vi "HFRR ADV v07 new software.vi"() -> ()   [LabVIEW 2025] (continued)
        n796 = local write "LIVE FEED MAX TEMP"(TRUE ("LIVE FEED MAX TEMP")) -> ()
        n797 = case shown="True" w1177 {
          selector: w1177 -> [_ w1186]
          frame False {
          }
          frame True {
            n798 = Not(x=w1186) -> (.not. x?=w1185:bool)
            n799 = local write "LIVE FEED MIN TEMP"(w1185) -> ()
            n800 = call "CAMERA LIVE FEED FGV.vi"("Enum - Menu"=CAMERA_LIVE_FEED_ENUM."CAMERA MINIMIZE") -> ()  [unwired: 9 in, 2 out]
          }
        }
        n801 = case shown="True" w1175 {
          selector: w1175 -> [_ w1183]
          frame False {
          }
          frame True {
            n802 = Not(x=w1183) -> (.not. x?=w1181:bool)
            n803 = local write "CAMERA ROI MAX TEMP"(w1181) -> ()
            n804 = call "IMAGE ANALYSIS.vi"("Enum"=POST_ANALYSIS_ENUM."SHOW UI") -> ("error out"=w1180:errorcluster)  [unwired: 9 in, 1 out]
            n805 = call "LIST FILE NAMES.vi"("error in (no error)"=w1180) -> ("filenames"=w1179:string[])  [unwired: 9 in, 1 out]
            n806 = property on="Test File List :" class="CmbBox"("Strings[]"=w1179) -> ()  [unwired: 2 in, 2 out]
          }
        }
        n807 = local write "CAMERA ROI MIN TEMP"(TRUE ("CAMERA ROI MIN TEMP")) -> ()
      }
      frame "Compare Files" {
        n808 = local read "LIVE FEED MIN TEMP"() -> (w1189:bool)
        n809 = local write "LIVE FEED MAX TEMP"(TRUE ("LIVE FEED MAX TEMP")) -> ()
        n810 = local read "CAMERA ROI MIN TEMP"() -> (w1187:bool)
        n811 = case shown="True" w1189 {
          selector: w1189 -> [_ w1196]
          frame False {
          }
          frame True {
            n812 = Not(x=w1196) -> (.not. x?=w1195:bool)
            n813 = local write "LIVE FEED MIN TEMP"(w1195) -> ()
            n814 = call "CAMERA LIVE FEED FGV.vi"("Enum - Menu"=CAMERA_LIVE_FEED_ENUM."CAMERA MINIMIZE") -> ()  [unwired: 9 in, 2 out]
          }
        }
        n815 = case shown="True" w1187 {
          selector: w1187 -> [_ w1193]
          frame False {
          }
          frame True {
            n816 = Not(x=w1193) -> (.not. x?=w1192:bool)
            n817 = local write "CAMERA ROI MIN TEMP"(w1192) -> ()
            n818 = call "IMAGE ANALYSIS.vi"("Enum"=POST_ANALYSIS_ENUM."MINIMIZE UI") -> ()  [unwired: 9 in, 2 out]
          }
        }
        n819 = local write "CAMERA ROI MAX TEMP"(TRUE ("CAMERA ROI MAX TEMP")) -> ()
      }
      frame "About" {
        n820 = local read "LIVE FEED MIN TEMP"() -> (w1199:bool)
        n821 = local write "LIVE FEED MAX TEMP"(TRUE ("LIVE FEED MAX TEMP")) -> ()
        n822 = local read "CAMERA ROI MIN TEMP"() -> (w1198:bool)
        n823 = case shown="True" w1199 {
          selector: w1199 -> [_ w1206]
          frame False {
          }
          frame True {
            n824 = Not(x=w1206) -> (.not. x?=w1205:bool)
            n825 = local write "LIVE FEED MIN TEMP"(w1205) -> ()
            n826 = call "CAMERA LIVE FEED FGV.vi"("Enum - Menu"=CAMERA_LIVE_FEED_ENUM."CAMERA MINIMIZE") -> ()  [unwired: 9 in, 2 out]
          }
        }
        n827 = case shown="True" w1198 {
          selector: w1198 -> [_ w1203]
          frame False {
          }
          frame True {
            n828 = Not(x=w1203) -> (.not. x?=w1202:bool)
            n829 = local write "CAMERA ROI MIN TEMP"(w1202) -> ()
            n830 = call "IMAGE ANALYSIS.vi"("Enum"=POST_ANALYSIS_ENUM."MINIMIZE UI") -> ()  [unwired: 9 in, 2 out]
          }
        }
        n831 = local write "CAMERA ROI MAX TEMP"(TRUE ("CAMERA ROI MIN TEMP")) -> ()
      }
      frame "Advance" {
        n832 = local read "LIVE FEED MIN TEMP"() -> (w1209:bool)
        n833 = local write "LIVE FEED MAX TEMP"(TRUE ("LIVE FEED MAX TEMP")) -> ()
        n834 = local read "CAMERA ROI MIN TEMP"() -> (w1207:bool)
        n835 = case shown="True" w1209 {
          selector: w1209 -> [_ w1216]
          frame False {
          }
          frame True {
            n836 = Not(x=w1216) -> (.not. x?=w1215:bool)
            n837 = local write "LIVE FEED MIN TEMP"(w1215) -> ()
            n838 = call "CAMERA LIVE FEED FGV.vi"("Enum - Menu"=CAMERA_LIVE_FEED_ENUM."CAMERA MINIMIZE") -> ()  [unwired: 9 in, 2 out]
          }
        }
        n839 = local write "CAMERA ROI MAX TEMP"(TRUE ("CAMERA ROI MAX TEMP")) -> ()
        n840 = case shown="True" w1207 {
          selector: w1207 -> [_ w1213]
          frame False {
          }
          frame True {
            n841 = Not(x=w1213) -> (.not. x?=w1212:bool)
            n842 = local write "CAMERA ROI MIN TEMP"(w1212) -> ()
            n843 = call "IMAGE ANALYSIS.vi"("Enum"=POST_ANALYSIS_ENUM."MINIMIZE UI") -> ()  [unwired: 9 in, 2 out]
          }
        }
      }
      frame "Mooha" {
        n844 = local read "LIVE FEED MIN TEMP"() -> (w1219:bool)
        n845 = local write "LIVE FEED MAX TEMP"(TRUE ("LIVE FEED MAX TEMP")) -> ()
        n846 = local read "CAMERA ROI MIN TEMP"() -> (w1217:bool)
        n847 = case shown="True" w1219 {
          selector: w1219 -> [_ w1226]
          frame False {
          }
          frame True {
            n848 = Not(x=w1226) -> (.not. x?=w1225:bool)
            n849 = local write "LIVE FEED MIN TEMP"(w1225) -> ()
            n850 = call "CAMERA LIVE FEED FGV.vi"("Enum - Menu"=CAMERA_LIVE_FEED_ENUM."CAMERA MINIMIZE") -> ()  [unwired: 9 in, 2 out]
          }
        }
        n851 = local write "CAMERA ROI MAX TEMP"(TRUE ("CAMERA ROI MAX TEMP")) -> ()
        n852 = case shown="True" w1217 {
          selector: w1217 -> [_ w1223]
          frame False {
          }
          frame True {
            n853 = Not(x=w1223) -> (.not. x?=w1222:bool)
            n854 = local write "CAMERA ROI MIN TEMP"(w1222) -> ()
            n855 = call "IMAGE ANALYSIS.vi"("Enum"=POST_ANALYSIS_ENUM."MINIMIZE UI") -> ()  [unwired: 9 in, 2 out]
          }
        }
      }
    }
    n856 = local read "Auto Start Test"() -> (w963:bool)
    n857 = case shown="True" "sign in temp" {
      frame False {
      }
      frame True {
        w999 = 1 ("y")
        n858 = local read "USERNAME"() -> (w1005:string)
        n859 = local read "USER ID"() -> (w1002:string)
        n860 = call <vilib>:"Trim Whitespace.vi"("string"=w1005) -> ("trimmed string"=w1004:string)  [unwired: 1 in]
        n861 = call <vilib>:"Trim Whitespace.vi"("string"=w1002) -> ("trimmed string"=w1003:string)  [unwired: 1 in]
        n862 = String Length(string=w1004) -> (length=w1001:i32)
        n863 = String Length(string=w1003) -> (length=w1000:i32)
        n864 = Greater?(x=w1001, y=w999) -> (0:w998:bool)
        n865 = Greater?(x=w1000, y=w999) -> (0:w997:bool)
        n866 = And(x=w998, y=w997) -> (x .and. y?=w996:bool)
        n867 = case shown="True" w996 {
          frame False {
            n868 = property on="Sign In" class="Bool (strict)"("DisabledEnum"=T15."Disabled" ("Disabled")) -> ()  [unwired: 2 in, 2 out]
          }
          frame True {
            n869 = property on="Sign In" class="Bool (strict)"("DisabledEnum"=T15."Enabled" ("Disabled")) -> ()  [unwired: 2 in, 2 out]
          }
        }
      }
    }
    n870 = local read "Air Temperature"() -> (w980:bool)
    n871 = local read "Coefficient Of Friction"() -> (w981:bool)
    n872 = case shown="False" w963 {
      frame False {
        n873 = local read "Auto stop temp"() -> (w993:bool)
        n874 = case shown="True" w993 {
          frame False {
          }
          frame True {
            n875 = local write "Auto Start Temp"(FALSE ("Auto Start Temp")) -> ()
          }
        }
      }
      frame True {
        "Auto stop temp" <- TRUE ("Auto stop temp")
      }
    }
    n876 = local read "Humidity"() -> (w979:bool)
    n877 = case shown="\"HOME\"" w990 {
      frame "HOME" {
        n878 = local write "main tab sub"(enum32{"Page 1", "Page 2"}."Page 1" ("main tab sub")) -> ()
      }
      frame Default {
        n879 = local write "main tab sub"(enum32{"Page 1", "Page 2"}."Page 2" ("main tab sub")) -> ()
      }
    }
    n880 = case shown="True" w989 {
      selector: w989 -> [_ w1332]
      frame False {
      }
      frame True {
        n881 = Not(x=w1332) -> (.not. x?=w1331:bool)
        n882 = local write "Sign In"(w1331) -> ()
        n883 = local write "Main Dashboard Buttons"(T21."Test Setup" ("Main Dashboard Buttons")) -> ()
      }
    }
    n884 = case shown="\"Numeric Display\", Default" "Num/Graph" {
      frame "Numeric Display", Default {
        n885 = property on="Single/Multiple" class="RadioBtnsControl (strict)"("Visible"=FALSE) -> ()  [unwired: 2 in, 2 out]
        n886 = property on="Single - Graph" class="Ring (strict)"("Visible"=FALSE) -> ()  [unwired: 2 in, 2 out]
        n887 = local write "Main Tab Display"(T4."Dashboard 1" ("Main Tab Display")) -> ()
      }
      frame "Graph Display" {
        n888 = property on="Single/Multiple" class="RadioBtnsControl (strict)"("Visible"=TRUE) -> ()  [unwired: 2 in, 2 out]
        n889 = case shown="\"Multiple\"" "Single/Multiple" {
          frame "Single ", Default {
            n890 = property on="Single - Graph" class="Ring (strict)"("Visible"=TRUE) -> ()  [unwired: 2 in, 2 out]
            n891 = local write "Main Tab Display"(T4."Dashboard 3" ("Main Tab Display")) -> ()
          }
          frame "Multiple" {
            n892 = property on="Single - Graph" class="Ring (strict)"("Visible"=FALSE) -> ()  [unwired: 2 in, 2 out]
            n893 = local write "Main Tab Display"(T4."Dashboard 2" ("Main Tab Display")) -> ()
          }
        }
      }
    }
    n894 = local read "Stroke"() -> (w978:bool)
    n895 = local read "USERNAME"() -> (w984:string)
    n896 = local read "USER ID"() -> (w983:string)
    n897 = case shown="True" w981 {
      selector: w981 -> [_ w1266]
      frame False {
      }
      frame True {
        n898 = Not(x=w1266) -> (.not. x?=w1265:bool)
        n899 = local write "Coefficient Of Friction"(w1265) -> ()
        n900 = local write "Tab Control 2"(T6."Coefficient Of Friction" ("Tab Control 2")) -> ()
      }
    }
    n901 = case shown="True" w980 {
      selector: w980 -> [_ w1263]
      frame False {
      }
      frame True {
        n902 = Not(x=w1263) -> (.not. x?=w1261:bool)
        n903 = local write "Air Temperature"(w1261) -> ()
        n904 = local write "Tab Control 2"(T6."Air Temperature" ("Tab Control 2")) -> ()
      }
    }
    n905 = local write "Operator ID"(w983) -> ()
    n906 = case shown="True" w978 {
      selector: w978 -> [_ w1257]
      frame False {
      }
      frame True {
        n907 = Not(x=w1257) -> (.not. x?=w1255:bool)
        n908 = local write "Stroke"(w1255) -> ()
        n909 = local write "Tab Control 2"(T6."Stroke" ("Tab Control 2")) -> ()
      }
    }
    n910 = local write "tested by"(w984) -> ()
    n911 = case shown="True" w979 {
      selector: w979 -> [_ w1260]
      frame False {
      }
      frame True {
        n912 = Not(x=w1260) -> (.not. x?=w1258:bool)
        n913 = local write "Humidity"(w1258) -> ()
        n914 = local write "Tab Control 2"(T6."Humidity" ("Tab Control 2")) -> ()
      }
    }
    n915 = case shown="\"Calibration\"" "Main Dashboard Buttons" {
      tunnel: [T2."HOME" ("Main Tab") T2."Test Setup" ("Main Tab") T2."Acquire" ("Main Tab") T2."Adv Scar" ("Main Tab") T2."Adv Scar Report" ("Main Tab") T2."Compare Files" ("Main Tab") T2."Calibration" ("Main Tab") T2."About" ("Main Tab") T2."Advance" ("Main Tab")] -> w962
      frame "Home", Default {
      }
      frame "Test Setup" {
      }
      frame "Dashboard" {
      }
      frame "Imaging" {
      }
      frame "Report" {
      }
      frame "Analysis" {
      }
      frame "Calibration" {
      }
      frame "About" {
      }
      frame "Advance" {
      }
    }
    n916 = Wait (ms)(milliseconds to wait=u32 100) -> ()  [unwired: 1 out]
    n917 = local read "Main Tab Display"() -> (w982:T4)
    n918 = local write "Main Tab"(w962) -> ()
    n919 = case shown="\"Dashboard 3\"" w982 {
      frame "Dashboard 1", Default {
        n920 = property on="Reset Graph" class="Bool (strict)"("Visible"=FALSE) -> ()  [unwired: 2 in, 2 out]
      }
      frame "Dashboard 2" {
        n921 = property on="Reset Graph" class="Bool (strict)"("Visible"=TRUE) -> ()  [unwired: 2 in, 2 out]
      }
      frame "Dashboard 3" {
        n922 = property on="Reset Graph" class="Bool (strict)"("Visible"=TRUE) -> ()  [unwired: 2 in, 2 out]
      }
    }
    n923 = local read "SCAR MEASURMENT"() -> (w970:enum32{"Auto Scar", "Manual Scar"})
    n924 = local read "Humidity"() -> (w985:bool)
    n925 = local read "Cap Live Image"() -> (w967:bool)
    n926 = local read "Sample Temperature"() -> (w977:bool)
    n927 = local read "Air Temp vs Humidity"() -> (w975:bool)
    n928 = local read "Frequency"() -> (w976:bool)
    n929 = case shown="False" w985 {
      frame False {
        n930 = local write "Humidity On Command"(TRUE ("Humidity On Command")) -> ()
        n931 = case shown="True" "Humidity Off Command" {
          selector: "Humidity Off Command" -> [_ w1273]
          frame False {
          }
          frame True {
            n932 = stacked-sequence {
              frame #0 {
                n933 = local read "WriteHumidity"() -> (w1275:string[])
                n934 = Insert Into Array(array=w1275, new element="R;1" ("new element/subarray")) -> (w1276:string[])  [unwired: 1 in]
                n935 = local write "WriteHumidity"(w1276) -> ()
              }
              frame #1 {
                n936 = Wait (ms)(milliseconds to wait=u32 2000) -> ()  [unwired: 1 out]
              }
              frame #2 {
                n937 = local read "EVENT LOG"() -> (w1282:string)
                n938 = local read "WriteHumidity"() -> (w1279:string[])
                n939 = call "Event Log.vi"("Content"="Humidity Control Off" ("string"), "EVENT LOG"=w1282) -> ("EVENT LOG"=w1283:string)  [unwired: 8 in, 1 out]
                n940 = local write "EVENT LOG"(w1283) -> ()
                n941 = Insert Into Array(array=w1279, new element="R;1" ("new element/subarray")) -> (w1280:string[])  [unwired: 1 in]
                n942 = local write "WriteHumidity"(w1280) -> ()
              }
            }
            n943 = Not(x=w1273) -> (.not. x?=w1272:bool)
            n944 = local write "Humidity Off Command"(w1272) -> ()
          }
        }
      }
      frame True {
        n945 = local write "Humidity Off Command"(TRUE ("Humidity Off Command")) -> ()
        n946 = case shown="False" "Humidity On Command" {
          selector: "Humidity On Command" -> [_ w1287]
          frame False {
          }
          frame True {
            n947 = stacked-sequence {
              frame #0 {
                n948 = local read "Set Rh"() -> (w1293:dbl)
                n949 = Number To Fractional String(number=w1293, precision (6)=i16 2) -> (F-format string=w1294:string)  [unwired: 2 in]
                n950 = local read "WriteHumidity"() -> (w1291:string[])
                n951 = Concatenate Strings("M;" ("new element/subarray"), w1294) -> (w1292:string)
                n952 = Insert Into Array(array=w1291, new element=w1292) -> (w1290:string[])  [unwired: 1 in]
                n953 = local write "WriteHumidity"(w1290) -> ()
              }
              frame #1 {
                n954 = Wait (ms)(milliseconds to wait=u32 1500) -> ()  [unwired: 1 out]
              }
              frame #2 {
                (unwired) "% RH" ("string")
                (unwired) i16 2 ("precision (6)")
                (unwired) "M;" ("new element/subarray")
                n955 = local read "Set Rh"() -> (w1301:dbl)
                n956 = Number To Fractional String(number=w1301, precision (6)=i16 2) -> (F-format string=w1298:string)  [unwired: 2 in]
                n957 = local read "WriteHumidity"() -> (w1303:string[])
                n958 = Concatenate Strings("M;" ("new element/subarray"), w1298) -> (w1302:string)
                n959 = Concatenate Strings("Humidity Set to : " ("string"), w1298, "% RH" ("string")) -> (w1296:string)
                n960 = Insert Into Array(array=w1303, new element=w1302) -> (w1304:string[])  [unwired: 1 in]
                n961 = disable-structure shown="Enabled" {
                  frame Enabled {
                    n962 = local read "EVENT LOG"() -> (w1307:string)
                    n963 = call "Event Log.vi"("Content"="Humidity Control On", "EVENT LOG"=w1307) -> ("EVENT LOG"=w1308:string)  [unwired: 8 in, 1 out]
                    n964 = local write "EVENT LOG"(w1308) -> ()
                  }
                  frame Disabled {
                  }
                }
                n965 = disable-structure shown="Enabled" {
                  disable-tunnel: w1296 -> [_ _]
                  frame Enabled {
                    n966 = local read "EVENT LOG"() -> (w1310:string)
                    n967 = call "Event Log.vi"("Content"="Humidity Control On", "EVENT LOG"=w1310) -> ("EVENT LOG"=w1311:string)  [unwired: 8 in, 1 out]
                    n968 = local write "EVENT LOG"(w1311) -> ()
                  }
                  frame Disabled {
                  }
                }
                n969 = local write "WriteHumidity"(w1304) -> ()
              }
            }
            n970 = Not(x=w1287) -> (.not. x?=w1286:bool)
            n971 = local write "Humidity On Command"(w1286) -> ()
          }
        }
      }
    }
    n972 = Equal?(x=w970, y=enum32{"Auto Scar", "Manual Scar"}."Auto Scar" ("SCAR MEASURMENT")) -> (x = y?=w966:bool)
    n973 = local read "TEST STANDARD"() -> (w973:T3)
    n974 = And(x=w967, y=w966) -> (x .and. y?=w968:bool)
    n975 = case shown="True" w968 {
      selector: w968 -> [_ w1072]
      tunnel: errorcluster {"status"=FALSE, "code"=0, "source"=""} ("error in (no error) 3") -> [_ w1073]
      frame False {
      }
      frame True {
        n976 = stacked-sequence {
          tunnel: w1073 -> [_ _ _ _ _ _ _ w1121]
          tunnel: w1072 -> [_ _ _ _ _ w1102 _ _]
          frame #0 {
            n977 = call "CAMERA LIVE FEED FGV.vi"("Enum - Menu"=CAMERA_LIVE_FEED_ENUM."CAMERA MINIMIZE") -> ()  [unwired: 9 in, 2 out]
          }
          frame #1 {
            n978 = property on="Auto Scar Check  2" class="Clust (strict)"("Visible"=TRUE) -> ()  [unwired: 2 in, 2 out]
          }
          frame #2 {
            n979 = String To Path(string="C:\\LAB-IQ\\Image Calibrate v01.dcf") -> (path=w1078:path)
            n980 = Open/Create/Replace File ("Open File")(file path (use dialog)=w1078) -> (refnum out=w1079:refnum<file>)  [unwired: 5 in, 2 out]
            n981 = for {
              N: 4 -> [_]
              tunnel: w1079 -> [w1085]
              i -> [w1081]
              n982 = Read from Text File ("Read File")(file (use dialog)=w1085) -> (text=w1086:string)  [unwired: 3 in, 3 out]
              n983 = String Subset(string=w1086, offset (0)=6, length (rest)=10 ("length (rest)")) -> (substring=w1082:string)
              n984 = Fract/Exp String To Number(string=w1082) -> (number=w1080:dbl)  [unwired: 3 in, 1 out]
              n985 = case shown="0" w1081 {
                tunnel: w1080 -> [w1087 w1088 _ w1089 _]
                frame 0 {
                  "5x Gain" <- w1087
                }
                frame 1 {
                  "10x Gain" <- w1088
                }
                frame 2 {
                }
                frame 3 {
                  "100x gain" <- w1089
                }
                frame 4, Default {
                }
              }
            }
          }
          frame #3 {
            n986 = local read "FILE 3"() -> (w1095:string)
            n987 = call <vilib>:"Trim Whitespace.vi"("string"="C:\\LAB-IQ\\images\\") -> ("trimmed string"=w1097:string)  [unwired: 1 in]
            n988 = String To Path(string=w1097) -> (path=w1096:path)
            n989 = Concatenate Strings(w1095, ".png" ("string")) -> (w1094:string)
            n990 = Build Path(base path=w1096, name or relative path=w1094) -> (appended path=w1092:path)
            "Image path" <- w1092
            n991 = Path To String(path=w1092) -> (string=w1091:string)
            n992 = call "CAMERA LIVE FEED FGV.vi"("Enum - Menu"=CAMERA_LIVE_FEED_ENUM."CAMERA SAVE", "Image Path"=w1091) -> ()  [unwired: 8 in, 2 out]
          }
          frame #4 {
            n993 = One Button Dialog(message="Image saved successfully") -> ()  [unwired: 1 in, 1 out]
          }
          frame #5 {
            n994 = local read "TEST STANDARD"() -> (w1101:T3)
            n995 = local read "Magnification len live scar"() -> (w1113:string)
            n996 = Not(x=w1102) -> (.not. x?=w1103:bool)
            n997 = local write "Cap Live Image"(w1103) -> ()
            n998 = case shown="\"ISO 12156\"" w1101 {
              tunnel: ["ASTM D6079" "ISO 12156"] -> w1100
              frame "ASTM D6079", Default {
              }
              frame "ISO 12156" {
              }
            }
            n999 = case shown="\"5x\", Default" w1113 {
              tunnel: [w1116 w1117] -> w1112
              frame "5x", Default {
                n1000 = local read "5x Gain"() -> (w1116:dbl)
              }
              frame "10x" {
                # "5x"
                n1001 = local read "10x Gain"() -> (w1117:dbl)
              }
            }
            n1002 = local read "Image path"() -> (w1111:path)
            n1003 = local read "FILE 3"() -> (w1104:string)
            n1004 = call "EDGE DETCTION.vi"("GAIN VALUE"=w1112, "Image Path"=w1111) -> ("error out"=w1110:errorcluster, "return value"=w1109:cluster{string, string, dbl, dbl, dbl})  [unwired: 8 in]
            n1005 = Bundle By Name(cluster=T22 {"File Name"="", "Test Method"="", "Operator"="", "Fuel Description"="", "Date and time"=""} ("Main Ref"), "File Name"=w1104, "Test Method"=w1100) -> (w1105:T22)
            n1006 = call "duf file read.vi"("error in (no error)"=w1110, "Main Ref"=w1105) -> ("error out"=w1108:errorcluster, "Main Ref 2"=w1106:T22)  [unwired: 8 in]
            n1007 = call "EDGE DETECTION REPORT.vi"("error in (no error)"=w1108, "return value 2"=w1109, "Main Ref"=w1106) -> ()  [unwired: 8 in, 1 out]
          }
          frame #6 {
            n1008 = property on="Auto Scar Check  2" class="Clust (strict)"("Visible"=FALSE) -> ()  [unwired: 2 in, 2 out]
          }
          frame #7 {
            n1009 = call "CAMERA LIVE FEED FGV.vi"("Enum - Menu"=CAMERA_LIVE_FEED_ENUM."CAMERA MINIMIZE", "error in (no error)"=w1121) -> ()  [unwired: 8 in, 2 out]
            n1010 = local write "Main Dashboard Buttons"(T1."Home" ("Main Dashboard Buttons")) -> ()
            n1011 = local write "Main Tab"(T2."HOME" ("Main Tab")) -> ()
          }
        }
      }
    }
    n1012 = local read "Heater Button"() -> (w974:bool)
    n1013 = case shown="True" w976 {
      selector: w976 -> [_ w1251]
      frame False {
      }
      frame True {
        n1014 = Not(x=w1251) -> (.not. x?=w1249:bool)
        n1015 = local write "Frequency"(w1249) -> ()
        n1016 = local write "Tab Control 2"(T6."Frequency" ("Tab Control 2")) -> ()
      }
    }
    n1017 = case shown="True" w975 {
      selector: w975 -> [_ w1248]
      frame False {
      }
      frame True {
        n1018 = Not(x=w1248) -> (.not. x?=w1246:bool)
        n1019 = local write "Air Temp vs Humidity"(w1246) -> ()
        n1020 = local write "Tab Control 2"(T6."Air Temp vs Rh" ("Tab Control 2")) -> ()
      }
    }
    n1021 = case shown="True" w977 {
      selector: w977 -> [_ w1254]
      frame False {
      }
      frame True {
        n1022 = Not(x=w1254) -> (.not. x?=w1252:bool)
        n1023 = local write "Sample Temperature"(w1252) -> ()
        n1024 = local write "Tab Control 2"(T6."Sample Temperature" ("Tab Control 2")) -> ()
      }
    }
    n1025 = case shown="\"Custom\"" w973 {
      frame "ASTM D6079", Default {
        w1227 = "ASTM D6079 TEST CONDITIONS" ("Standard 2")
        n1026 = local write "Standard 2"(w1227) -> ()
        n1027 = local write "Standard"(w1227) -> ()
      }
      frame "ISO 12156" {
        w1228 = "ISO 12156 TEST CONDITIONS" ("Standard 2")
        n1028 = local write "Standard 2"(w1228) -> ()
        n1029 = local write "Standard"(w1228) -> ()
      }
      frame "CEC F-096-A-06" {
        w1229 = "CEC F-096-A-06 TEST CONDITIONS" ("Standard 2")
        n1030 = local write "Standard 2"(w1229) -> ()
        n1031 = local write "Standard"(w1229) -> ()
      }
      frame "Custom" {
        w1230 = "CUSTOM TEST CONDITIONS" ("Standard 2")
        n1032 = local write "Standard 2"(w1230) -> ()
        n1033 = local write "Standard"(w1230) -> ()
      }
    }
    n1034 = case shown="True" w974 {
      frame False {
        n1035 = local write "Temperature On Command"(TRUE ("Temperature On Command")) -> ()
        n1036 = case shown="True" "Temperature Off Command" {
          selector: "Temperature Off Command" -> [_ w1234]
          frame False {
          }
          frame True {
            n1037 = Not(x=w1234) -> (.not. x?=w1233:bool)
            n1038 = local read "EVENT LOG"() -> (w1237:string)
            n1039 = local write "Temperature Off Command"(w1233) -> ()
            n1040 = call "Event Log.vi"("Content"="Heater Off", "EVENT LOG"=w1237) -> ("EVENT LOG"=w1236:string)  [unwired: 8 in, 1 out]
            n1041 = local write "EVENT LOG"(w1236) -> ()
          }
        }
      }
      frame True {
        n1042 = local write "Temperature Off Command"(TRUE ("Temperature Off Command")) -> ()
        n1043 = case shown="True" "Temperature On Command" {
          selector: "Temperature On Command" -> [_ w1241]
          frame False {
          }
          frame True {
            n1044 = Not(x=w1241) -> (.not. x?=w1240:bool)
            n1045 = local write "Temperature On Command"(w1240) -> ()
            n1046 = disable-structure shown="Enabled" {
              disable-tunnel: "Heater On" -> [w1243 _]
              frame Enabled {
                n1047 = local read "EVENT LOG"() -> (w1244:string)
                n1048 = call "Event Log.vi"("Content"=w1243, "EVENT LOG"=w1244) -> ("EVENT LOG"=w1245:string)  [unwired: 8 in, 1 out]
                n1049 = local write "EVENT LOG"(w1245) -> ()
              }
              frame Disabled {
              }
            }
          }
        }
      }
    }
    n1050 = local read "Main Tab"() -> (w965:T2)
    n1051 = case shown="\"About\"" w965 {
      frame "HOME", Default {
        w1008 = T15."Enabled" ("Disabled")
        n1052 = local read "Service Password enable"() -> (w1010:bool)
        n1053 = property on="Imaging" class="Bool (strict)"("DisabledEnum"=w1008) -> ()  [unwired: 2 in, 2 out]
        n1054 = property on="Dashboard" class="Bool (strict)"("DisabledEnum"=w1008) -> ()  [unwired: 2 in, 2 out]
        n1055 = property on="Test Setup" class="Bool (strict)"("DisabledEnum"=w1008) -> ()  [unwired: 2 in, 2 out]
        n1056 = property on="Analysis" class="Bool (strict)"("DisabledEnum"=w1008) -> ()  [unwired: 2 in, 2 out]
        n1057 = property on="Home" class="Bool (strict)"("DisabledEnum"=w1008) -> ()  [unwired: 2 in, 2 out]
        n1058 = property on="Report" class="Bool (strict)"("DisabledEnum"=w1008) -> ()  [unwired: 2 in, 2 out]
        n1059 = property on="Main Dashboard Buttons" class="RadioBtnsControl (strict)"("DisabledEnum"=w1008) -> ()  [unwired: 2 in, 2 out]
        n1060 = property on="Calibration" class="Bool (strict)"("DisabledEnum"=w1008) -> ()  [unwired: 2 in, 2 out]
        n1061 = case shown="True" w1010 {
          tunnel: [T15."Disabled" ("Disabled") T15."Enabled" ("Disabled")] -> w1009
          frame False {
          }
          frame True {
          }
        }
        n1062 = property on="About" class="Bool (strict)"("DisabledEnum"=w1009) -> ()  [unwired: 2 in, 2 out]
      }
      frame "Test Setup" {
        w1015 = T15."Enabled" ("Disabled")
        n1063 = local read "Service Password enable"() -> (w1014:bool)
        n1064 = property on="Dashboard" class="Bool (strict)"("DisabledEnum"=T15."Disabled" ("Disabled")) -> ()  [unwired: 2 in, 2 out]
        n1065 = property on="Imaging" class="Bool (strict)"("DisabledEnum"=w1015) -> ()  [unwired: 2 in, 2 out]
        n1066 = property on="Analysis" class="Bool (strict)"("DisabledEnum"=w1015) -> ()  [unwired: 2 in, 2 out]
        n1067 = property on="Home" class="Bool (strict)"("DisabledEnum"=w1015) -> ()  [unwired: 2 in, 2 out]
        n1068 = property on="Report" class="Bool (strict)"("DisabledEnum"=w1015) -> ()  [unwired: 2 in, 2 out]
        n1069 = property on="Test Setup" class="Bool (strict)"("DisabledEnum"=w1015) -> ()  [unwired: 2 in, 2 out]
        n1070 = case shown="True" w1014 {
          tunnel: [T15."Disabled" ("Disabled") T15."Enabled" ("Disabled")] -> w1013
          frame False {
          }
          frame True {
          }
        }
        n1071 = property on="About" class="Bool (strict)"("DisabledEnum"=w1013) -> ()  [unwired: 2 in, 2 out]
      }
      frame "Adv Scar" {
        w1022 = T15."Enabled" ("Disabled")
        n1072 = property on="Dashboard" class="Bool (strict)"("DisabledEnum"=T15."Disabled" ("Disabled")) -> ()  [unwired: 2 in, 2 out]
        n1073 = property on="Imaging" class="Bool (strict)"("DisabledEnum"=w1022) -> ()  [unwired: 2 in, 2 out]
        n1074 = property on="Analysis" class="Bool (strict)"("DisabledEnum"=w1022) -> ()  [unwired: 2 in, 2 out]
        n1075 = property on="Home" class="Bool (strict)"("DisabledEnum"=w1022) -> ()  [unwired: 2 in, 2 out]
        n1076 = property on="Report" class="Bool (strict)"("DisabledEnum"=w1022) -> ()  [unwired: 2 in, 2 out]
        n1077 = property on="Test Setup" class="Bool (strict)"("DisabledEnum"=w1022) -> ()  [unwired: 2 in, 2 out]
        n1078 = local read "Service Password enable"() -> (w1020:bool)
        n1079 = case shown="True" w1020 {
          tunnel: [T15."Disabled" ("Disabled") T15."Enabled" ("Disabled")] -> w1019
          frame False {
          }
          frame True {
          }
        }
        n1080 = property on="About" class="Bool (strict)"("DisabledEnum"=w1019) -> ()  [unwired: 2 in, 2 out]
      }
      frame "Calibration" {
        w1025 = T15."Enabled" ("Disabled")
        n1081 = property on="Dashboard" class="Bool (strict)"("DisabledEnum"=T15."Disabled" ("Disabled")) -> ()  [unwired: 2 in, 2 out]
        n1082 = property on="Imaging" class="Bool (strict)"("DisabledEnum"=w1025) -> ()  [unwired: 2 in, 2 out]
        n1083 = property on="Analysis" class="Bool (strict)"("DisabledEnum"=w1025) -> ()  [unwired: 2 in, 2 out]
        n1084 = property on="Home" class="Bool (strict)"("DisabledEnum"=w1025) -> ()  [unwired: 2 in, 2 out]
        n1085 = property on="Report" class="Bool (strict)"("DisabledEnum"=w1025) -> ()  [unwired: 2 in, 2 out]
        n1086 = property on="Test Setup" class="Bool (strict)"("DisabledEnum"=w1025) -> ()  [unwired: 2 in, 2 out]
        n1087 = local read "Service Password enable"() -> (w1027:bool)
        n1088 = property on="Calibration" class="Bool (strict)"("DisabledEnum"=w1025) -> ()  [unwired: 2 in, 2 out]
        n1089 = case shown="True" w1027 {
          tunnel: [T15."Disabled" ("Disabled") T15."Enabled" ("Disabled")] -> w1026
          frame False {
          }
          frame True {
          }
        }
        n1090 = property on="About" class="Bool (strict)"("DisabledEnum"=w1026) -> ()  [unwired: 2 in, 2 out]
      }
      frame "Adv Scar Report" {
        w1033 = T15."Enabled" ("Disabled")
        n1091 = property on="Dashboard" class="Bool (strict)"("DisabledEnum"=T15."Disabled" ("Disabled")) -> ()  [unwired: 2 in, 2 out]
        n1092 = property on="Imaging" class="Bool (strict)"("DisabledEnum"=w1033) -> ()  [unwired: 2 in, 2 out]
        n1093 = property on="Analysis" class="Bool (strict)"("DisabledEnum"=w1033) -> ()  [unwired: 2 in, 2 out]
        n1094 = property on="Home" class="Bool (strict)"("DisabledEnum"=w1033) -> ()  [unwired: 2 in, 2 out]
        n1095 = property on="Report" class="Bool (strict)"("DisabledEnum"=w1033) -> ()  [unwired: 2 in, 2 out]
        n1096 = property on="Test Setup" class="Bool (strict)"("DisabledEnum"=w1033) -> ()  [unwired: 2 in, 2 out]
        n1097 = local read "Service Password enable"() -> (w1032:bool)
        n1098 = case shown="True" w1032 {
          tunnel: [T15."Disabled" ("Disabled") T15."Enabled" ("Disabled")] -> w1031
          frame False {
          }
          frame True {
          }
        }
        n1099 = property on="About" class="Bool (strict)"("DisabledEnum"=w1031) -> ()  [unwired: 2 in, 2 out]
      }
      frame "Compare Files" {
        w1039 = T15."Enabled" ("Disabled")
        n1100 = local read "Service Password enable"() -> (w1038:bool)
        n1101 = property on="Dashboard" class="Bool (strict)"("DisabledEnum"=T15."Disabled" ("Disabled")) -> ()  [unwired: 2 in, 2 out]
        n1102 = property on="Imaging" class="Bool (strict)"("DisabledEnum"=w1039) -> ()  [unwired: 2 in, 2 out]
        n1103 = property on="Analysis" class="Bool (strict)"("DisabledEnum"=w1039) -> ()  [unwired: 2 in, 2 out]
        n1104 = property on="Home" class="Bool (strict)"("DisabledEnum"=w1039) -> ()  [unwired: 2 in, 2 out]
        n1105 = property on="Report" class="Bool (strict)"("DisabledEnum"=w1039) -> ()  [unwired: 2 in, 2 out]
        n1106 = property on="Test Setup" class="Bool (strict)"("DisabledEnum"=w1039) -> ()  [unwired: 2 in, 2 out]
        n1107 = case shown="True" w1038 {
          tunnel: [T15."Disabled" ("Disabled") T15."Enabled" ("Disabled")] -> w1037
          frame False {
          }
          frame True {
          }
        }
        n1108 = property on="About" class="Bool (strict)"("DisabledEnum"=w1037) -> ()  [unwired: 2 in, 2 out]
      }
      frame "Acquire" {
        n1109 = local read "Service Password enable"() -> (w1044:bool)
        n1110 = property on="Test Setup" class="Bool (strict)"("DisabledEnum"=T15."Disabled" ("Disabled")) -> ()  [unwired: 2 in, 2 out]
        n1111 = local read "Auto Start Test"() -> (w1046:bool)
        n1112 = local read "RUN"() -> (w1048:bool)
        n1113 = case shown="True" w1044 {
          tunnel: [T15."Disabled" ("Disabled") T15."Enabled" ("Disabled")] -> w1045
          frame False {
          }
          frame True {
          }
        }
        n1114 = Or(x=w1048, y=w1046) -> (x .or. y?=w1047:bool)
        n1115 = case shown="True" w1047 {
          tunnel: [T15."Enabled" ("Disabled") T15."Disabled" ("Disabled")] -> w1043
          frame False {
          }
          frame True {
          }
        }
        n1116 = property on="About" class="Bool (strict)"("DisabledEnum"=w1045) -> ()  [unwired: 2 in, 2 out]
        n1117 = property on="Imaging" class="Bool (strict)"("DisabledEnum"=w1043) -> ()  [unwired: 2 in, 2 out]
        n1118 = property on="Dashboard" class="Bool (strict)"("DisabledEnum"=w1043) -> ()  [unwired: 2 in, 2 out]
        n1119 = property on="Analysis" class="Bool (strict)"("DisabledEnum"=w1043) -> ()  [unwired: 2 in, 2 out]
        n1120 = property on="Home" class="Bool (strict)"("DisabledEnum"=w1043) -> ()  [unwired: 2 in, 2 out]
        n1121 = property on="Report" class="Bool (strict)"("DisabledEnum"=w1043) -> ()  [unwired: 2 in, 2 out]
        n1122 = property on="Calibration" class="Bool (strict)"("DisabledEnum"=w1043) -> ()  [unwired: 2 in, 2 out]
      }
      frame "About" {
        n1123 = local read "FILE"() -> (w1062:string)
        n1124 = local read "TEST FILE NAM,E SAVED"() -> (w1055:bool)
        n1125 = call <vilib>:"Trim Whitespace.vi"("string"=w1062) -> ("trimmed string"=w1061:string)  [unwired: 1 in]
        n1126 = local read "Auto Start Test"() -> (w1065:bool)
        n1127 = String Length(string=w1061) -> (length=w1060:i32)
        n1128 = Greater?(x=w1060, y=1) -> (0:w1057:bool)
        n1129 = And(x=w1057, y=w1055) -> (x .and. y?=w1056:bool)
        n1130 = local read "RUN"() -> (w1067:bool)
        n1131 = case shown="True" w1056 {
          tunnel: [T15."Disabled" ("Disabled") T15."Enabled" ("Disabled")] -> w1058
          frame False {
          }
          frame True {
          }
        }
        n1132 = Or(x=w1067, y=w1065) -> (x .or. y?=w1066:bool)
        n1133 = property on="About" class="Bool (strict)"("DisabledEnum"=T15."Enabled" ("Disabled")) -> ()  [unwired: 2 in, 2 out]
        n1134 = case shown="False" w1066 {
          tunnel: [T15."Enabled" ("Disabled") T15."Disabled" ("Disabled")] -> w1064
          frame False {
          }
          frame True {
          }
        }
        n1135 = property on="Dashboard" class="Bool (strict)"("DisabledEnum"=w1058) -> ()  [unwired: 2 in, 2 out]
        n1136 = property on="Test Setup" class="Bool (strict)"("DisabledEnum"=T15."Disabled" ("Disabled")) -> ()  [unwired: 2 in, 2 out]
        n1137 = property on="Imaging" class="Bool (strict)"("DisabledEnum"=w1064) -> ()  [unwired: 2 in, 2 out]
        n1138 = property on="Analysis" class="Bool (strict)"("DisabledEnum"=w1064) -> ()  [unwired: 2 in, 2 out]
        n1139 = property on="Home" class="Bool (strict)"("DisabledEnum"=w1064) -> ()  [unwired: 2 in, 2 out]
        n1140 = property on="Report" class="Bool (strict)"("DisabledEnum"=w1064) -> ()  [unwired: 2 in, 2 out]
      }
    }
    n1141 = local read "Quit"() -> (w992:bool)
    "Single" <- "Single - Graph"
  }
  n1142 = disable-structure shown="Disabled" {
    disable-tunnel: [w1336 _] -> w39
    disable-tunnel: _ -> [w1335 _]
    frame Disabled {
      n1143 = while {
        tunnel: w1335 -> [_]
        tunnel: [w1337] -> w1336
        tunnel: [w1338] -> _
        i -> [w1338]
        stop <- w1337 stop-if-true
        w1354 = u16 10 items=["1.0"=10, "1.5"=15, "2.0"=20] ("stop bits (10: 1 bit)")
        n1144 = Wait (ms)(milliseconds to wait=u32 10) -> ()  [unwired: 1 out]
        n1145 = call-poly "VISA Configure Serial Port"("VISA resource name"=refnum<visa-resource-name> "ASRL1::INSTR" ("COM PORT"), "timeout (10sec)"=u32 10, "baud rate (9600)"=u32 57600, "data bits (8)"=u16 8, "stop bits (10: 1 bit)"=w1354) -> ("VISA resource name out"=w1340:refnum<visa-resource-name>, "error out"=w1349:errorcluster)  [unwired: 9 in]
        n1146 = VISA Read(VISA resource name=w1340, byte count=u32 2 ("byte count (0)")) -> (read buffer=w1348:string)  [unwired: 1 in, 3 out]
        n1147 = String Subset(string=w1348, offset (0)=0, length (rest)=2 ("length (rest)")) -> (substring=w1347:string)
        n1148 = Match Pattern(string=w1347, regular expression="<>") -> (offset past match=w1344:i32)  [unwired: 1 in, 3 out]
        n1149 = Greater Or Equal?(x=w1344, y=0) -> (x >= y?=w1339:bool)
        n1150 = case shown="True" w1339 {
          tunnel: w1340 -> [_ w1358]
          tunnel: w1349 -> [_ w1357]
          frame False {
          }
          frame True {
            n1151 = VISA Read(VISA resource name=w1358, byte count=u32 32 ("byte count (0)"), error in (no error)=w1357) -> (read buffer=w1356:string)  [unwired: 3 out]
            n1152 = String Subset(string=w1356, offset (0)=0, length (rest)=8 ("length (rest)")) -> (substring=w1360:string)
            n1153 = String Subset(string=w1356, offset (0)=8, length (rest)=8 ("length (rest)")) -> (substring=w1361:string)
            n1154 = Decimal String To Number(string=w1361) -> (number=w1368:i32)  [unwired: 2 in, 1 out]
            n1155 = Decimal String To Number(string=w1360) -> (number=w1364:i32)  [unwired: 2 in, 1 out]
            n1156 = Divide(x=w1368, y=10000) -> ()  [unwired: 1 out]
            n1157 = Divide(x=w1364, y=1000000) -> ()  [unwired: 1 out]
          }
        }
        n1158 = local read "Quit"() -> (w1337:bool)
      }
    }
    frame Enabled {
    }
  }
  n1159 = while {
    shift-right: [w1383] -> w52
    shift-left: _ -> [w1374]
    shift-right: [w1382] -> w51
    shift-left: errorcluster {"status"=TRUE, "code"=0, "source"="Init"} ("error IO") -> [w1376]
    tunnel: [w1371] -> w42
    tunnel: [w1381] -> _
    i -> [w1381]
    stop <- w1371 stop-if-true
    n1160 = local read "Port 1a"() -> (w1377:bool)
    n1161 = local read "Port 3"() -> (w1378:bool)
    n1162 = local read "Com Port 1"() -> (w1375:refnum<visa-resource-name>)
    n1163 = Or(x=w1378, y=w1377) -> (x .or. y?=w1380:bool)
    n1164 = Unbundle(w1376) -> ("status"=→"Port 3":bool)  [unwired: 2 out]
    n1165 = Not Equal?(x=w1375, y=w1374) -> (x != y?=w1372:bool)
    n1166 = case shown="True" w1380 {
      frame False {
        w1386 = TRUE ("Visible")
        n1167 = property on="Port 1a" class="Bool (strict)"("Visible"=w1386) -> ()  [unwired: 2 in, 2 out]
        n1168 = property on="Port 3" class="Bool (strict)"("Visible"=w1386) -> ()  [unwired: 2 in, 2 out]
      }
      frame True {
        w1387 = TRUE ("Visible")
        n1169 = property on="Port 1a" class="Bool (strict)"("Visible"=w1387) -> ()  [unwired: 2 in, 2 out]
        n1170 = property on="Port 3" class="Bool (strict)"("Visible"=w1387) -> ()  [unwired: 2 in, 2 out]
      }
    }
    n1171 = Wait (ms)(milliseconds to wait=u32 40) -> ()  [unwired: 1 out]
    n1172 = case shown="True" w1372 {
      tunnel: [w1384 errorcluster {"status"=TRUE, "code"=0, "source"="Init"} ("error out")] -> w1373
      tunnel: w1376 -> [w1384 _]
      frame False {
      }
      frame True {
      }
    }
    n1173 = case shown="Error" w1373 {
      selector: w1373 -> [w1395 w1422]
      tunnel: [w1389 w1426] -> w1383
      tunnel: [w1397 w1420] -> w1382
      tunnel: w1374 -> [w1396 w1424]
      frame No Error {
        n1174 = property class="Instr"(reference=w1396, error in=w1395) -> (reference out=w1393:refnum<visa-resource-name>, error out=w1394:errorcluster, "Serial Settings:Number of Bytes at Serial Port"=w1390:u32)
        n1175 = Greater?(x=w1390, y=u32 5) -> (0:w1388:bool)
        n1176 = Not(x=w1388) -> (.not. x?=→"Port 1a":bool)
        n1177 = while {
          tunnel: [w1415] -> w1397
          tunnel: [w1414] -> w1398
          tunnel: w1394 -> [w1413]
          tunnel: w1393 -> [w1412]
          stop <- TRUE stop-if-true
          n1178 = property class="Instr" props=["Serial Settings:Number of Bytes at Serial Port"](reference=w1412, error in=w1413) -> (reference out=w1417:refnum<visa-resource-name>, error out=w1416:errorcluster)  [unwired: 1 out]
          n1179 = VISA Read(VISA resource name=w1417, byte count=u32 50, error in (no error)=w1416) -> (VISA resource name out=w1414:refnum<visa-resource-name>, read buffer=w1399:string, error out=w1415:errorcluster)  [unwired: 1 out]
          "UNI READ" <- w1399
          n1180 = Spreadsheet String To Array(delimiter (Tab)=";", format string="", spreadsheet string=w1399, array type (2D Dbl)=dbl[] []) -> (array=w1409:dbl[])
          n1181 = Index Array(array=w1409) -> (element #1=→"LVDT MIN":dbl, element #2=→"LVDT MAX":dbl, element #3=→"LVDT Peak":dbl, element #4=→"pizo raw":dbl, element #5=→"Friction":dbl, element #6=→"cof 2":dbl)  [unwired: 6 in]
        }
        n1182 = VISA Flush I/O Buffer(VISA resource name=w1398) -> (VISA resource name out=w1389:refnum<visa-resource-name>)  [unwired: 2 in, 1 out]
      }
      frame Error {
        w1432 = u16 0 items=["None", "XON/XOFF", "RTS/CTS", "XON/XOFF & RTS/CTS", "DTR/DSR", "XON/XOFF & DTR/DSR"] ("flow control (0:none)  2")
        w1430 = u16 10 items=["1.0"=10, "1.5"=15, "2.0"=20] ("stop bits 2")
        w1428 = u16 0 items=["None", "Odd", "Even", "Mark", "Space"] ("parity 2")
        w1429 = u32 10000  # timeout (10sec)
        n1183 = VISA Close(VISA resource name=w1424, error in (no error)=w1422) -> (error out=w1425:errorcluster)
        n1184 = local write "Port 1a"(FALSE ("Port 1a")) -> ()
        n1185 = local read "Com Port 1"() -> (w1419:refnum<visa-resource-name>)
        n1186 = call <vilib>:"Clear Errors.vi"("error in (no error)"=w1425) -> ("error out"=w1423:errorcluster)  [unwired: 5 in, 1 out]
        n1187 = call-poly "VISA Configure Serial Port"("VISA resource name"=w1419, "timeout (10sec)"=w1429, "baud rate (9600)"=u32 250000 ("baud rate  2"), "data bits (8)"=u16 8 ("data bits  2"), "parity (0:none)"=w1428, "error in (no error)"=w1423, "stop bits (10: 1 bit)"=w1430, "flow control (0:none)"=w1432) -> ("VISA resource name out"=w1433:refnum<visa-resource-name>, "error out"=w1434:errorcluster)  [unwired: 6 in]
        n1188 = flat-sequence {
          tunnel: w1433 -> [w1436]
          tunnel: w1434 -> [w1435]
          tunnel: [w1436] -> w1426
          tunnel: [w1435] -> w1420
          frame #0 {
            n1189 = Wait (ms)(milliseconds to wait=u32 50) -> ()  [unwired: 1 out]
          }
        }
        "Residual Uno" <- ""
        "Port 1 Error" <- w1420
      }
    }
    n1190 = local read "Quit"() -> (w1371:bool)
    "Error Uno" <- w1376
  }
  n1191 = while {
    stop <- w1443 stop-if-true
    # "V0OLTAGE TO STROKE (peice vise calibration)"
    n1192 = Wait (ms)(milliseconds to wait=u32 10) -> ()  [unwired: 1 out]
    n1193 = local read "LVDT Peak"() -> (w1440:dbl)
    n1194 = formula code="// Dynamic Parameterized Linear Interpolation Node\n// Inputs: vpp_val, voltages (Array), distances (Array)\n// Outputs: stroke\n\nint i = 0;\nint segments = 11; // 12 points make 11 interpolation segments\n\n// 1. Lower Boundary Clamp\nif (vpp_val <= voltages[0]) {\n    stroke = distances[0];\n}\n// 2. Upper Boundary Clamp\nelse if (vpp_val >= voltages[segments]) {\n    stroke = distances[segments];\n}\n// 3. Dynamic Segment Search Loop\nelse {\n    stroke = distances[0]; // Fallback baseline\n    for (i = 0; i < segments; i++) {\n        if (vpp_val >= voltages[i] && vpp_val <= voltages[i+1]) {\n            // Standard linear interpolation formula using array lookups\n            stroke = distances[i] + (vpp_val - voltages[i]) * (distances[i+1] - distances[i]) / (voltages[i+1] - voltages[i]);\n            break; // Segment found, safely exit the loop\n        }\n    }\n}"("vpp_val"=w1440, "voltages"="calibration values", "distances"="STROKE") -> ("stroke"=→"LVDT STROKE":dbl)
    n1195 = local read "Quit"() -> (w1443:bool)
  }
  n1196 = while {
    stop <- w1463 stop-if-true
    n1197 = call <vilib>:"High Resolution Polling Wait.vi"("seconds to wait"=0.02) -> ()  [unwired: 10 in, 1 out]
    n1198 = local read "Due read"() -> (w1461:string)
    n1199 = Spreadsheet String To Array(delimiter (Tab)=";", format string="", spreadsheet string=w1461, array type (2D Dbl)=string[] []) -> (array=w1458:string[])
    n1200 = Fract/Exp String To Number(string=w1458) -> (number=w1457:dbl[])  [unwired: 3 in, 1 out]
    n1201 = Index Array(array=w1457) -> (element #1=→"Sample Temperature":dbl, element #2=→"Target Sample Temperature":dbl, element #3=→"Current Duty Cycle":dbl, element #4=→"Ambient Temperature":dbl, element #5=→"Dac Status":dbl, element #6=→"Vpp":dbl, element #7=→"Active Error Code":dbl, element #8=→"Kp":dbl, element #9=→"Ki":dbl, element #10=→"Kd":dbl, element #11=→"SampleRaw":dbl, element #12=→"AmbRaw":dbl)  [unwired: 12 in]
    n1202 = local read "Quit"() -> (w1463:bool)
  }
  n1203 = while {
    shift-right: [w1477] -> w37
    shift-left: _ -> [w1468]
    shift-right: [w1476] -> w36
    shift-left: errorcluster {"status"=FALSE, "code"=0, "source"="Init"} ("error out") -> [w1470]
    tunnel: [w1465] -> w41
    tunnel: [w1475] -> _
    i -> [w1475]
    stop <- w1465 stop-if-true
    n1204 = local read "Com Port 2"() -> (w1469:refnum<visa-resource-name>)
    n1205 = local read "Port 2a"() -> (w1471:bool)
    n1206 = Unbundle(w1470) -> ("status"=→"Port 4":bool)  [unwired: 2 out]
    n1207 = call <vilib>:"High Resolution Polling Wait.vi"("seconds to wait"=0.02) -> ()  [unwired: 10 in, 1 out]
    n1208 = local read "Port 4"() -> (w1472:bool)
    n1209 = Not Equal?(x=w1469, y=w1468) -> (x != y?=w1467:bool)
    n1210 = Or(x=w1472, y=w1471) -> (x .or. y?=w1474:bool)
    n1211 = case shown="False" w1474 {
      frame False {
        w1480 = TRUE ("Visible")
        n1212 = property on="Port 2a" class="Bool (strict)"("Visible"=w1480) -> ()  [unwired: 2 in, 2 out]
        n1213 = property on="Port 4" class="Bool (strict)"("Visible"=w1480) -> ()  [unwired: 2 in, 2 out]
      }
      frame True {
        w1481 = TRUE ("Visible")
        n1214 = property on="Port 2a" class="Bool (strict)"("Visible"=w1481) -> ()  [unwired: 2 in, 2 out]
        n1215 = property on="Port 4" class="Bool (strict)"("Visible"=w1481) -> ()  [unwired: 2 in, 2 out]
      }
    }
    n1216 = case shown="True" w1467 {
      tunnel: [w1478 errorcluster {"status"=TRUE, "code"=0, "source"="Init"} ("error out")] -> w1466
      tunnel: w1470 -> [w1478 _]
      frame False {
      }
      frame True {
      }
    }
    n1217 = case shown="No Error" w1466 {
      selector: w1466 -> [w1492 w1523]
      tunnel: [w1485 w1528] -> w1477
      tunnel: [w1493 w1521] -> w1476
      tunnel: w1468 -> [w1495 w1526]
      frame No Error {
        n1218 = property class="Instr" props=["Serial Settings:Number of Bytes at Serial Port"](reference=w1495, error in=w1492) -> (reference out=w1486:refnum<visa-resource-name>, error out=w1491:errorcluster)  [unwired: 1 out]
        n1219 = while {
          tunnel: [w1503] -> w1487
          tunnel: [w1502] -> w1488
          tunnel: w1491 -> [w1501]
          tunnel: w1486 -> [w1500]
          tunnel: [w1499] -> _
          i -> [w1499]
          stop <- TRUE stop-if-true
          n1220 = property class="Instr" props=["Serial Settings:Number of Bytes at Serial Port"](reference=w1500, error in=w1501) -> (reference out=w1505:refnum<visa-resource-name>, error out=w1504:errorcluster)  [unwired: 1 out]
          n1221 = VISA Read(VISA resource name=w1505, byte count=u32 1000, error in (no error)=w1504) -> (VISA resource name out=w1502:refnum<visa-resource-name>, read buffer=→"Due read":string, error out=w1503:errorcluster)  [unwired: 1 out]
        }
        n1222 = local read "Command"() -> (w1483:string)
        n1223 = call <vilib>:"Trim Whitespace.vi"("string"=w1483) -> ("trimmed string"=w1482:string)  [unwired: 1 in]
        n1224 = Not Equal?(x=w1482, y="") -> (x != y?=w1489:bool)
        n1225 = case shown="True" w1489 {
          tunnel: w1488 -> [w1507 w1512]
          tunnel: [w1507 w1516] -> w1494
          tunnel: w1487 -> [w1506 w1511]
          tunnel: [w1506 w1514] -> w1493
          tunnel: w1482 -> [_ w1510]
          tunnel: [_ w1513] -> _
          frame False {
            # "DATA  WRITE LOOP"
          }
          frame True {
            n1226 = Concatenate Strings(w1510, "\r\n") -> (w1509:string)
            n1227 = VISA Write(VISA resource name=w1512, write buffer=w1509, error in (no error)=w1511) -> (VISA resource name out=w1516:refnum<visa-resource-name>, return count=w1513:u32, error out=w1515:errorcluster)
            n1228 = flat-sequence {
              tunnel: w1515 -> [w1518]
              tunnel: [w1518] -> w1514
              frame #0 {
                n1229 = local write "Command"("" ("Command")) -> ()
                n1230 = Wait (ms)(milliseconds to wait=u32 5) -> ()  [unwired: 1 out]
              }
            }
          }
        }
        n1231 = VISA Flush I/O Buffer(VISA resource name=w1494) -> (VISA resource name out=w1485:refnum<visa-resource-name>, error out=→"error out 9":errorcluster)  [unwired: 2 in]
      }
      frame Error {
        w1534 = u16 0 items=["None", "XON/XOFF", "RTS/CTS", "XON/XOFF & RTS/CTS", "DTR/DSR", "XON/XOFF & DTR/DSR"] ("flow control (0:none)  2")
        w1532 = u16 10 items=["1.0"=10, "1.5"=15, "2.0"=20] ("stop bits 2")
        w1530 = u16 0 items=["None", "Odd", "Even", "Mark", "Space"] ("parity 2")
        w1531 = u32 10000  # timeout (10sec)
        n1232 = VISA Clear(VISA resource name=w1526, error in (no error)=w1523) -> (VISA resource name out=w1525:refnum<visa-resource-name>, error out=w1524:errorcluster)
        n1233 = VISA Close(VISA resource name=w1525, error in (no error)=w1524) -> (error out=w1527:errorcluster)
        n1234 = call <vilib>:"Clear Errors.vi"("error in (no error)"=w1527) -> ()  [unwired: 5 in, 2 out]
        n1235 = local read "Com Port 2"() -> (w1520:refnum<visa-resource-name>)
        "visa due" <- w1520
        n1236 = call-poly "VISA Configure Serial Port"("VISA resource name"=w1520, "timeout (10sec)"=w1531, "baud rate (9600)"=u32 250000 ("baud rate  2"), "data bits (8)"=u16 8 ("data bits  2"), "parity (0:none)"=w1530, "stop bits (10: 1 bit)"=w1532, "flow control (0:none)"=w1534) -> ("VISA resource name out"=w1535:refnum<visa-resource-name>, "error out"=w1536:errorcluster)  [unwired: 7 in]
        n1237 = flat-sequence {
          tunnel: w1535 -> [w1538]
          tunnel: w1536 -> [w1537]
          tunnel: [w1538] -> w1528
          tunnel: [w1537] -> w1521
          frame #0 {
            n1238 = Wait (ms)(milliseconds to wait=u32 50) -> ()  [unwired: 1 out]
          }
        }
        "Residual Due" <- ""
        "Port 2 Error" <- w1521
      }
    }
    n1239 = local read "Quit"() -> (w1465:bool)
    "Error Due" <- w1470
  }
  n1240 = local write "FRICVALZ"(0.0 ("FRICVALZ")) -> ()
  n1241 = property on="RUN" class="Bool (strict)"("Visible"=TRUE) -> ()  [unwired: 2 in, 2 out]
  n1242 = while {
    tunnel: [w1555] -> _
    tunnel: [w1540] -> w54
    i -> [w1555]
    stop <- w1540 stop-if-true
    n1243 = local read "conststatus"() -> (w1544:dbl)
    n1244 = local read "Main Tab"() -> (w1542:T2)
    n1245 = local read "EDIT"() -> (w1561:bool)
    n1246 = local read "Rate"() -> (w1560:dbl)
    n1247 = case shown="True" w1561 {
      tunnel: [FALSE TRUE] -> w1547
      frame False {
      }
      frame True {
      }
    }
    n1248 = property on="Time slide" class="Slide (strict)"("Scale.Range:Maximum"=2500.0) -> ()  [unwired: 2 in, 2 out]
    n1249 = Equal?(x=w1542, y=T24."About" ("Main Tab")) -> (x = y?=w1553:bool)
    n1250 = Equal?(x=w1544, y=0.0) -> (x = y?=w1545:bool)
    n1251 = Divide(x=1.0, y=w1560) -> (x/y=w1556:dbl)
    "Time 2" <- w1556
    n1252 = case shown="True" w1545 {
      frame False {
      }
      frame True {
        # "C:\\WinDucom\\calibrate WO 2391.dcf"
        n1253 = local write "Lan flag"(22) -> ()
        n1254 = local write "conststatus"(10.0 ("rpm value : 2")) -> ()
        n1255 = String To Path(string="C:\\LAB-IQ\\calibrate WO 2465.dcf") -> (path=w1567:path)
        n1256 = Open/Create/Replace File "Open File"(file path (use dialog)=w1567) -> (refnum out=w1565:refnum<file>)  [unwired: 5 in, 2 out]
        n1257 = for {
          N: 23 -> [_]
          tunnel: w1565 -> [w1576]
          i -> [w1570]
          (unwired) TRUE ("line mode (F)")
          n1258 = Read from Text File "Read File"(file (use dialog)=w1576) -> (text=w1575:string)  [unwired: 3 in, 3 out]
          n1259 = Match Pattern(string=w1575, regular expression="]") -> (after substring=w1573:string)  [unwired: 1 in, 3 out]
          n1260 = String Subset(string=w1575, offset (0)=5, length (rest)=10 ("length (rest)")) -> (substring=w1568:string)
          n1261 = Fract/Exp String To Number(string=w1568) -> (number=w1569:dbl)  [unwired: 3 in, 1 out]
          n1262 = Match Pattern(string=w1573, regular expression="-") -> (before substring=w1571:string)  [unwired: 1 in, 3 out]
          n1263 = case shown="19" w1570 {
            tunnel: w1569 -> [w1579 w1580 w1581 w1582 _ _ _ w1587 w1588 _ w1589 w1590 w1591 w1592 w1593 w1594 _ w1595 w1596 _ _ _ _ _]
            tunnel: w1571 -> [_ _ _ _ w1583 w1584 w1585 _ _ _ _ _ _ _ _ _ _ _ _ w1597 w1598 w1599 w1600 _]
            frame 0 {
              n1264 = local write "FRIC. FORCE :"(w1579) -> ()
            }
            frame 1 {
              n1265 = local write "TEMPERATURE :"(w1580) -> ()
            }
            frame 2 {
              n1266 = local write "HUMIDITY:"(w1581) -> ()
            }
            frame 3 {
              n1267 = local write "AIR TEMPERATURE :"(w1582) -> ()
            }
            frame 4 {
              n1268 = local write "Com Port 1"(w1583) -> ()
            }
            frame 5 {
              n1269 = local write "Com Port 2"(w1584) -> ()
              n1270 = local write "visa due"(w1584) -> ()
            }
            frame 6 {
              n1271 = String To Path(string=w1585) -> (path=w1586:path)
              n1272 = local write "File Path"(w1586) -> ()
              "String" <- w1585
            }
            frame 7 {
              n1273 = local write "DISPLACEMENT :"(w1587) -> ()
            }
            frame 8 {
              n1274 = local write "STROKE GAIN :"(w1588) -> ()
            }
            frame 9 {
            }
            frame 10 {
